vi "test_riccat_03i.vi"() -> (3 "All Tests Passed":bool)   [LabVIEW 2019]
uses:
  <vilib>/Analysis/Matrix/Datatypes/RealMatrix.ctl
  <vilib>/Rock Robotics/WPI/ThirdParty/JAS_Junk/TrajLib/Trajectory_Library.lvlib
  <vilib>/Analysis/Matrix/NI_Matrix.lvlib
panel:
  out "error out 2":errorcluster
  out "Pos Semi Definite":bool
  out "Q_Chk_Passed":bool
  out "C":T1
  out "Q Check":T1
  out "Bad":bool
  out "Stable Bad":bool
  out "error out":errorcluster
  out "Eigenvalues":cdb[](array[numeric])
  out "Error":bool
  out "Iterations":i32
  out "Elapsed \nTime MS":dbl
  out "ZERO":T1
  out "X  Answer":T1
  in  "R":T1=[[1.0]]
  in  "Q":T1=[[1.0, 0.0], [0.0, 1.0]]
  in  "B":T1=[[0.0], [1.0]]
  in  "A":T1=[[0.0, 1.0], [0.0, 0.0]]
  # "// Test 3: the first generalized eigenvalue of (S,T) is stable"
  # "A3 << \n           0, 1, \n           0, 0;"
  # "B3 << \n0, \n1;"
  # "Q3 << \n      1, 0,\n      0, 1;"
  # "Example G2"
  # "Cost ??"
  # "R3 << 1;"
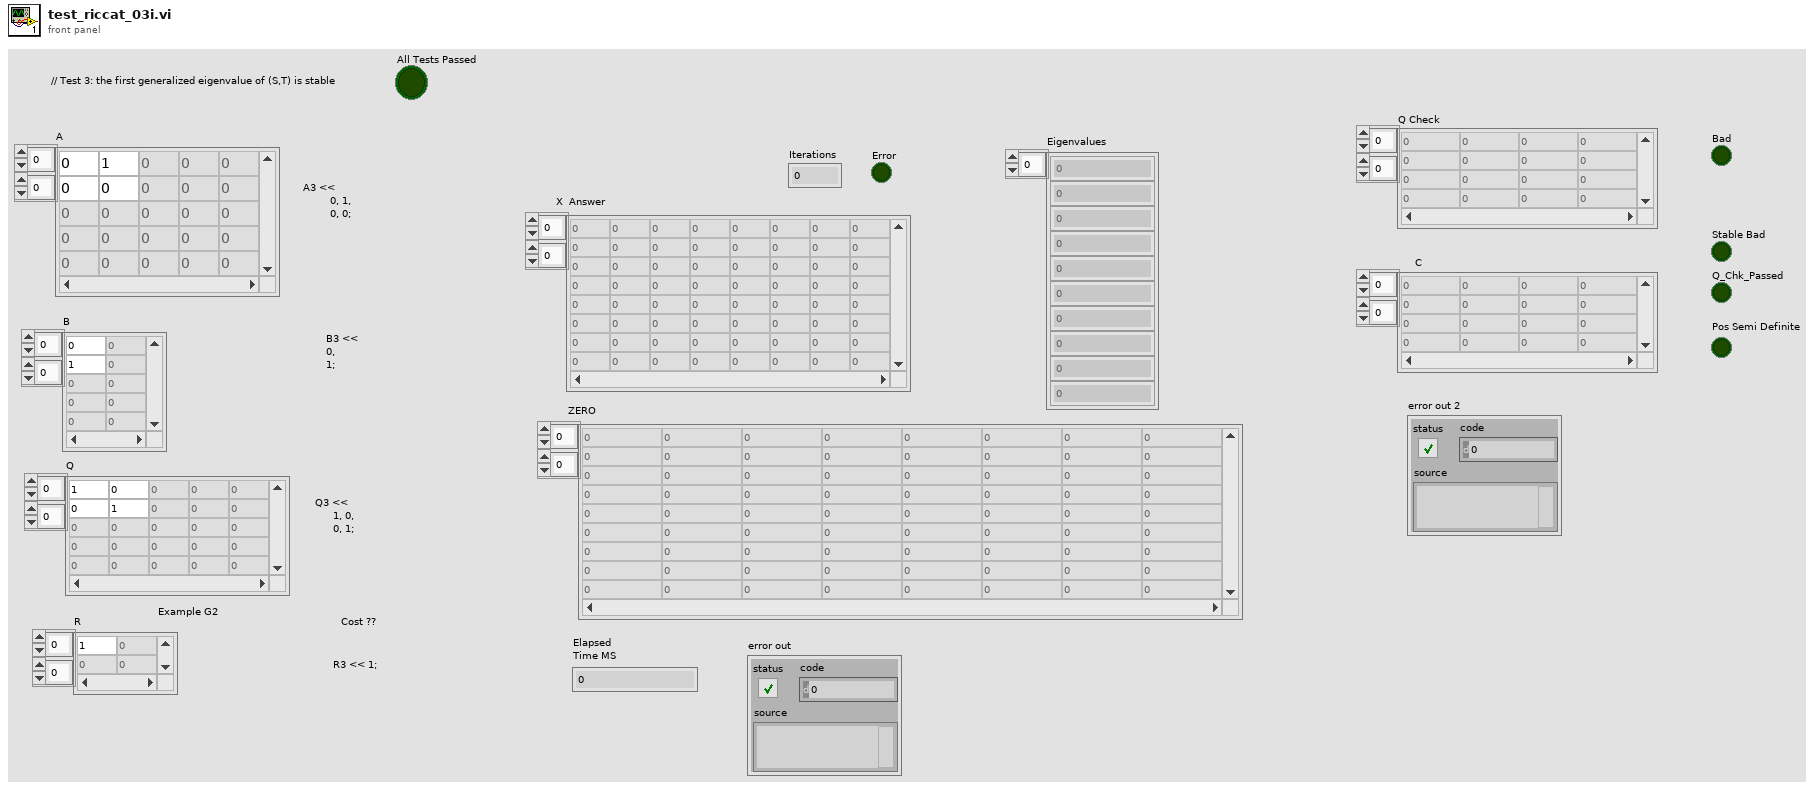
[diagram p1: front panel]
types:
  T1 = typedef "NI_Matrix.lvlib/RealMatrix.ctl" = dbl[][]
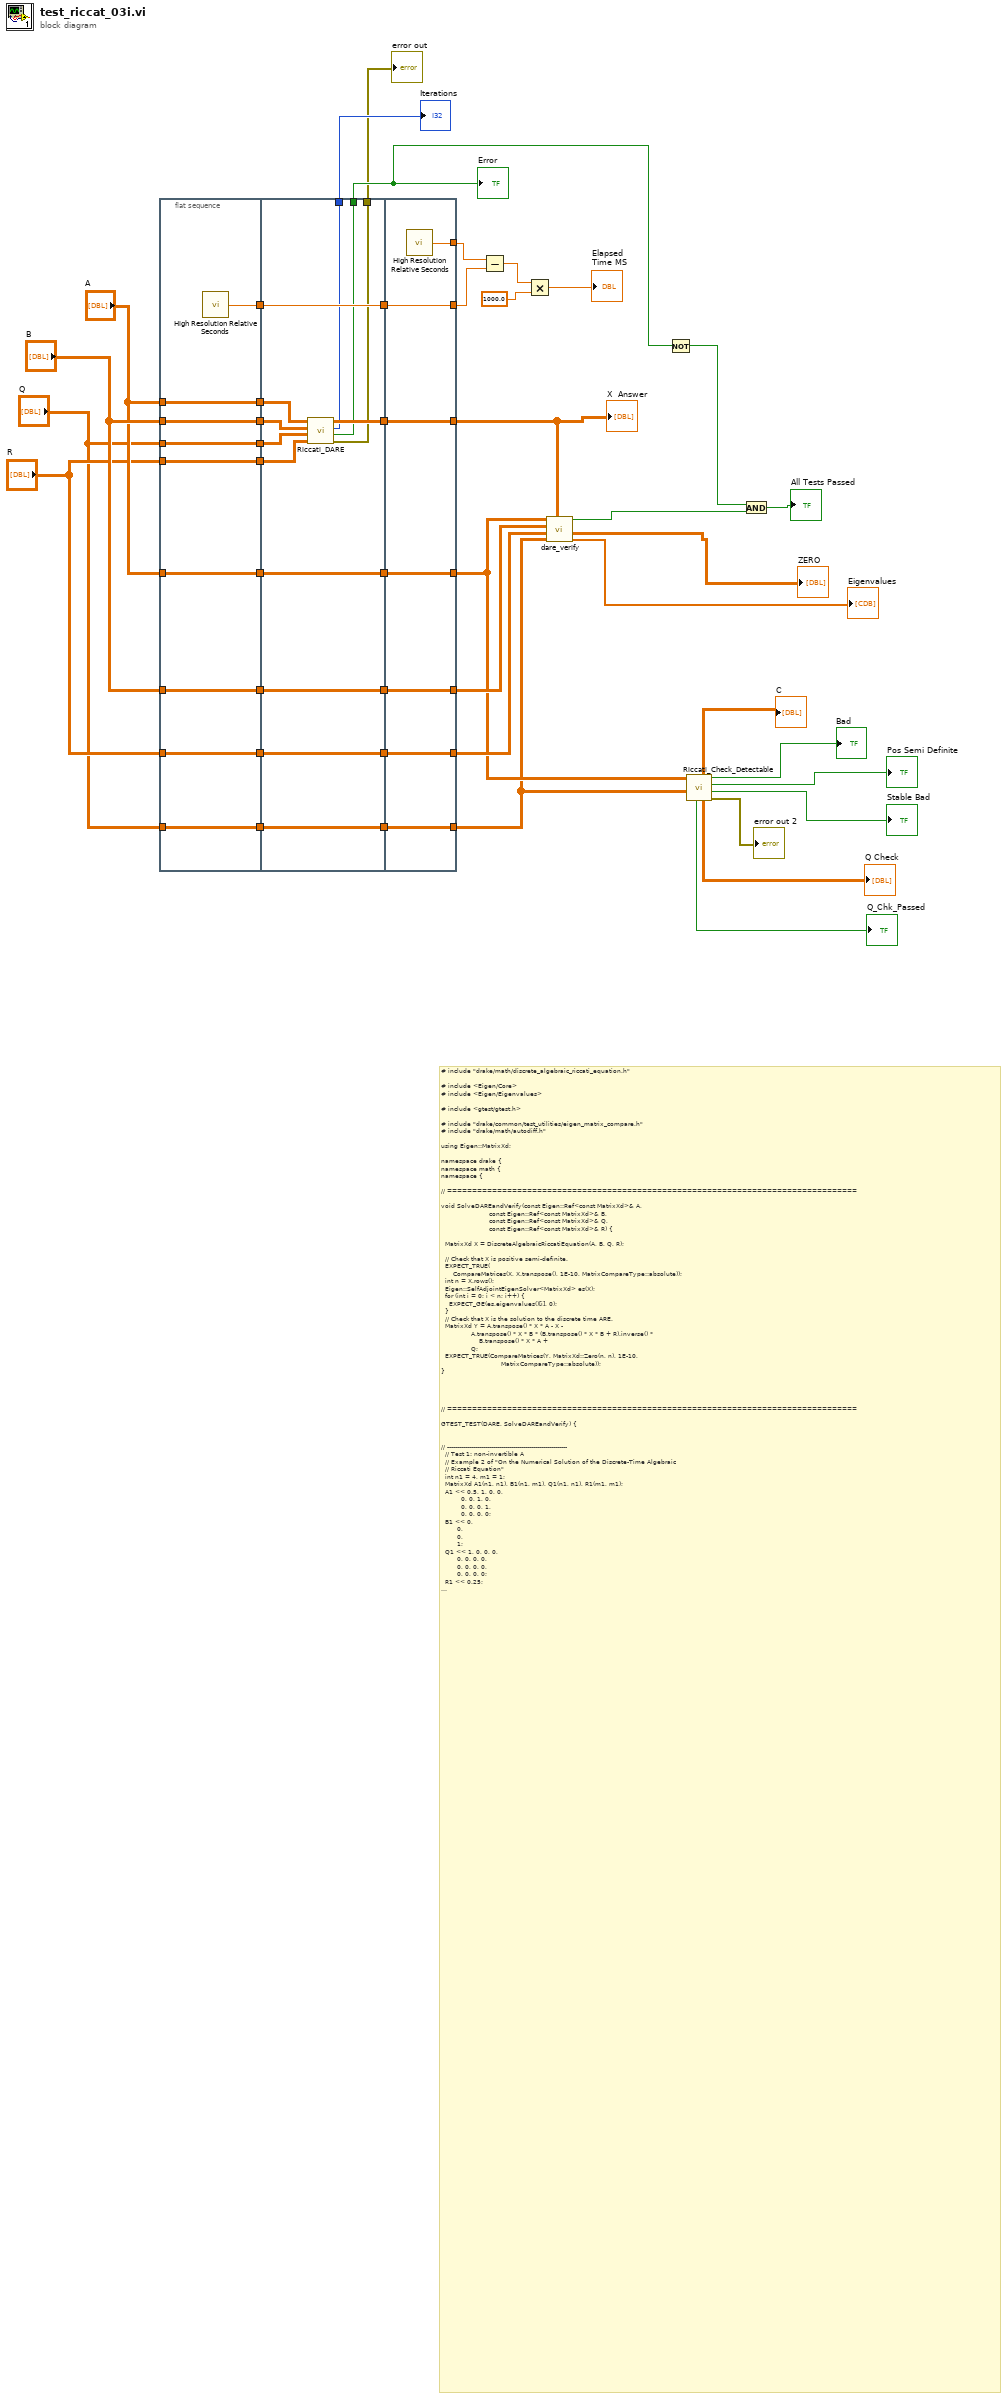
[diagram p0: block diagram]
diagram:
  # "# include \"drake/math/discrete_algebraic_riccati_equation.h\"\n\n# include <Eigen/Core>\n# include <Eigen/Eigenvalues>\n\n# include <gtest/gtest.h>\n\n# include \"drake/common/test_utilities/eigen_matrix_compare.h\"\n# include \"drake/math/autodiff.h\"\n\nusing Eigen::MatrixXd;\n\nnamespace drake {\nnamespace math {\nnamespace {\n\n// ==================================================================================\n\nvoid SolveDAREandVerify(const Eigen::Ref<const MatrixXd>& A,\n                        const Eigen::Ref<const MatrixXd>& B,\n                        const Eigen::Ref<const MatrixXd>& Q,\n                        const Eigen::Ref<const MatrixXd>& R) {\n\n  MatrixXd X = DiscreteAlgebraicRiccatiEquation(A, B, Q, R);\n\n  // Check that X is positive semi-definite.\n  EXPECT_TRUE(\n      CompareMatrices(X, X.transpose(), 1E-10, MatrixCompareType::absolute));\n  int n = X.rows();\n  Eigen::SelfAdjointEigenSolver<MatrixXd> es(X);\n  for (int i = 0; i < n; i++) {\n    EXPECT_GE(es.eigenvalues()[i], 0);\n  }\n  // Check that X is the solution to the discrete time ARE.\n  MatrixXd Y = A.transpose() * X * A - X -\n               A.transpose() * X * B * (B.transpose() * X * B + R).inverse() *\n                   B.transpose() * X * A +\n               Q;\n  EXPECT_TRUE(CompareMatrices(Y, MatrixXd::Zero(n, n), 1E-10,\n                              MatrixCompareType::absolute));\n}\n\n\n\n\n// ==================================================================================\n\nGTEST_TEST(DARE, SolveDAREandVerify) {\n\n\n// ------------------------------------------------------------\n  // Test 1: non-invertible A\n  // Example 2 of \"On the Numerical Solution of the Discrete-Time Algebraic\n  // Riccati Equation\"\n  int n1 = 4, m1 = 1;\n  MatrixXd A1(n1, n1), B1(n1, m1), Q1(n1, n1), R1(m1, m1);\n  A1 << 0.5, 1, 0, 0, \n          0, 0, 1, 0, \n          0, 0, 0, 1, \n          0, 0, 0, 0;\n  B1 << 0, \n        0, \n        0, \n        1;\n  Q1 << 1, 0, 0, 0, \n        0, 0, 0, 0, \n        0, 0, 0, 0, \n        0, 0, 0, 0;\n  R1 << 0.25;\n  SolveDAREandVerify(A1, B1, Q1, R1);\n// ------------------------------------------------------------\n  // Test 2: invertible A\n  int n2 = 2, m2 = 1;\n  MatrixXd A2(n2, n2), B2(n2, m2), Q2(n2, n2), R2(m2, m2);\n  A2 << 1, 1, 0, 1;\n  B2 << 0, 1;\n  Q2 << 1, 0, 0, 0;\n  R2 << 0.3;\n  SolveDAREandVerify(A2, B2, Q2, R2);\n\n// ------------------------------------------------------------\n  // Test 3: the first generalized eigenvalue of (S,T) is stable\n  int n3 = 2, m3 = 1;\n  MatrixXd A3(n3, n3), B3(n3, m3), Q3(n3, n3), R3(m3, m3);\n  A3 << 0, 1, 0, 0;\n  B3 << 0, 1;\n  Q3 << 1, 0, 0, 1;\n  R3 << 1;\n  SolveDAREandVerify(A3, B3, Q3, R3);\n\n// ------------------------------------------------------------\n  // Test 4: A = B = Q = R = I_2 (2-by-2 identity matrix)\n  int n4 = 2, m4 = 2;\n  MatrixXd A4(n4, n4), B4(n4, m4), Q4(n4, n4), R4(m4, m4);\n  A4 << 1, 0, 0, 1;\n  B4 << 1, 0, 0, 1;\n  Q4 << 1, 0, 0, 1;\n  R4 << 1, 0, 0, 1;\n  SolveDAREandVerify(A4, B4, Q4, R4);\n\n// ------------------------------------------------------------\n}\n}  // namespace\n}  // namespace math\n}  // namespace drake"
  n1 = flat-sequence {
    tunnel: "B" -> [w48]
    tunnel: "A" -> [w49]
    tunnel: "B" -> [w50]
    tunnel: "Q" -> [w51]
    tunnel: "A" -> [w52]
    tunnel: "R" -> [w53]
    tunnel: [w53] -> w44
    tunnel: [w52] -> w43
    tunnel: [w51] -> w42
    tunnel: [w50] -> w41
    tunnel: [w49] -> w40
    tunnel: [w48] -> w39
    tunnel: "R" -> [w47]
    tunnel: [w47] -> w32
    tunnel: "Q" -> [w46]
    tunnel: [w46] -> w30
    tunnel: [w45] -> w24
    tunnel: w44 -> [w66]
    tunnel: w43 -> [w64]
    tunnel: w42 -> [w63]
    tunnel: w41 -> [w62]
    tunnel: w40 -> [w61]
    tunnel: w39 -> [w60]
    tunnel: [w65] -> w38
    tunnel: [w61] -> w37
    tunnel: [w60] -> w36
    tunnel: [w59] -> w33
    tunnel: w32 -> [w59]
    tunnel: w30 -> [w58]
    tunnel: [w58] -> w29
    tunnel: [w57] -> w25
    tunnel: w24 -> [w57]
    tunnel: [w56] -> w20
    tunnel: [w55] -> w14
    tunnel: [w54] -> w10
    tunnel: [w71] -> w18
    tunnel: [w72] -> w7
    tunnel: [w73] -> w19
    tunnel: w38 -> [w73]
    tunnel: w37 -> [w72]
    tunnel: w36 -> [w71]
    tunnel: [w70] -> w17
    tunnel: w33 -> [w70]
    tunnel: [w69] -> w6
    tunnel: w29 -> [w69]
    tunnel: [w68] -> w27
    tunnel: [w67] -> w26
    tunnel: w25 -> [w67]
    frame #0 {
      n2 = call <vilib>:"High Resolution Relative Seconds.vi"() -> ("relative seconds"=w45:dbl)
    }
    frame #1 {
      n3 = call <vilib>:"Riccati_DARE.vi"("R"=w66, "Q"=w63, "B"=w62, "A"=w64) -> ("error out"=w54:errorcluster, "Error"=w55:bool, "Iterations"=w56:i32, "Answer"=w65:T1)  [unwired: 4 in]
    }
    frame #2 {
      n4 = call <vilib>:"High Resolution Relative Seconds.vi"() -> ("relative seconds"=w68:dbl)
    }
  }
  n5 = Subtract(x=w27, y=w26) -> (x-y=w23:dbl)
  n6 = Multiply(x=w23, y=1000.0) -> (x*y=→"Elapsed \nTime MS":dbl)
  n7 = call "dare_verify.vi"("Answer"=w19, "Q"=w6, "R"=w17, "B"=w18, "A"=w7) -> ("Eigenvalues"=→"Eigenvalues":cdb[], "ZERO"=→"ZERO":T1, "Passed"=w15:bool)  [unwired: 4 in]
  n8 = Not(x=w14) -> (.not. x?=w13:bool)
  n9 = call <vilib>:"Riccati_Check_Detectable.vi"("Q"=w6, "A"=w7) -> ("error out"=→"error out 2":errorcluster, "Stable Bad"=→"Stable Bad":bool, "Pos Semi Definite"=→"Pos Semi Definite":bool, "Bad"=→"Bad":bool, "Q_Check"=→"Q Check":T1, "C"=→"C":T1, "Q_Chk_Passed"=→"Q_Chk_Passed":bool)  [unwired: 3 in]
  n10 = And(x=w13, y=w15) -> (x .and. y?=→"All Tests Passed":bool)
  "X  Answer" <- w19
  "Iterations" <- w20
  "Error" <- w14
  "error out" <- w10
